vi "Find All Referenced Structures.vi"(8 "error in":errorcluster, 11 "ParseGDSII in":refnum<class "ParseGDSII.lvclass">) -> (0 "error out":errorcluster, 3 "ParseGDSII out":refnum<class "ParseGDSII.lvclass">)   [LabVIEW 2019, in "ParseGDSII.lvclass"]
uses:
  ParseGDSII.lvclass
  ParseGDSII.lvclass/ParseGDSII.ctl
  5fa63a74-4f9b-4856-8811-7cd17062abc4.vi
  DataTypes/Base/GDSII.DataType.lvclass
  Tree/Tree.lvclass
  Fast Tree/Fast Tree.lvclass
  920f742c-f628-416c-89cb-44049b089101.vi
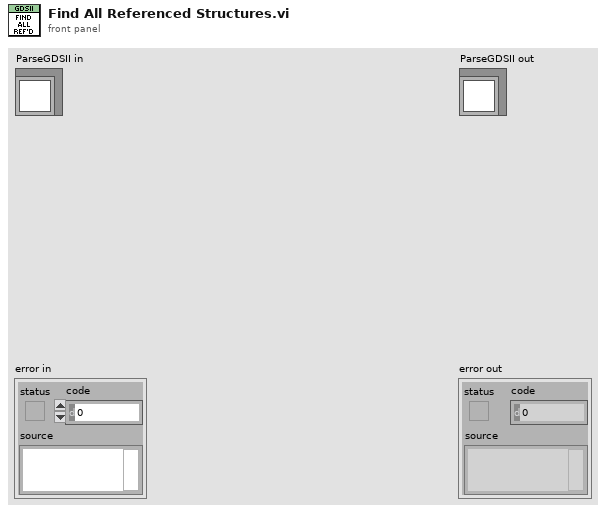
[diagram p1: front panel]
types:
  T1 = cluster{"Record Type":string, "Payload":string, "Parent Index":i32, "First Child Index":i32, "Next Sibling Index":i32}[]
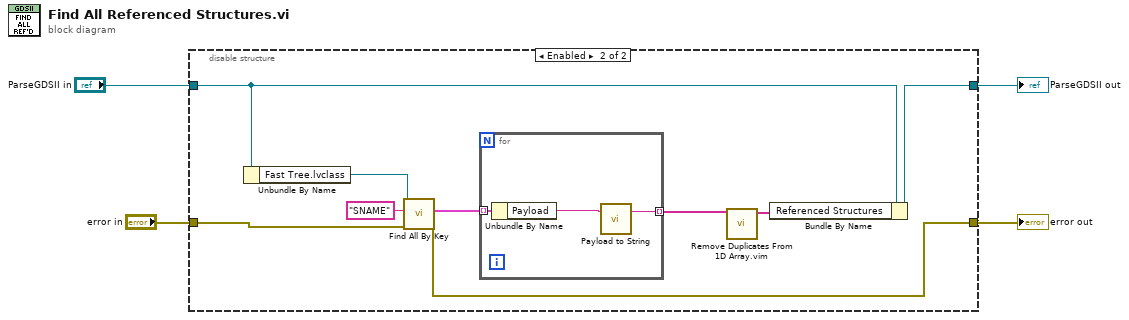
[diagram p0: block diagram]
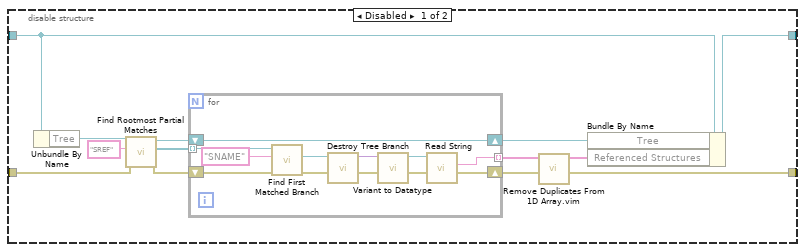
[diagram p2: hidden frame]
diagram:
  n1 = disable-structure shown="Enabled" {
    disable-tunnel: "error in" -> [w9 w28]
    disable-tunnel: [w8 w32] -> w3
    disable-tunnel: [w6 w30] -> w2
    disable-tunnel: "ParseGDSII in" -> [w5 w31]
    frame Disabled {
      n2 = Unbundle By Name(w5) -> ("Tree"=w12:refnum<class "Tree.lvclass">)
      n3 = call "Find Rootmost Partial Matches.vi"("error in"=w9, "Branch Name Pattern"="SREF", "Tree in"=w12) -> ("error out"=w10:errorcluster, "Root Most Partial Matches"=w14:refnum<class "Tree.lvclass">[], "Tree out"=w15:refnum<class "Tree.lvclass">)  [unwired: 5 in, 1 out]
      n4 = for {
        tunnel: w14 -> [w27] mode=indexing
        shift-right: [w22] -> w11
        shift-left: w15 -> [w22]
        tunnel: [w21] -> w13 mode=indexing
        shift-right: [w17] -> w8
        shift-left: w10 -> [w20]
        n5 = call "Find First Matched Branch.vi"("error in"=w20, "Branch Name Exact"="SNAME", "Tree in"=w27) -> ("error out"=w19:errorcluster, "Matched Branch"=w25:refnum<class "Tree.lvclass">)  [unwired: 5 in, 2 out]
        n6 = call "Destroy Tree Branch.vi"("error in"=w19, "Tree in"=w25) -> ("error out"=w18:errorcluster, "Root"=w24:variant)  [unwired: 8 in]
        n7 = call "Variant to Datatype.vi"("error in"=w18, "Variant"=w24) -> ("error out"=w17:errorcluster, "DataType"=w23:refnum<class "GDSII.DataType.lvclass">)  [unwired: 8 in]
        n8 = call-dynamic "Read String.vi"("GDSII.DataType in"=w23) -> ("String"=w21:string)  [unwired: 9 in, 1 out]
      }
      n9 = call "Remove Duplicates From 1D Array.vim"("array"=w13) -> ("array with duplicates removed"=w7:string[])  [unwired: 10 in]
      n10 = Bundle By Name(cluster=w5, "Tree"=w11, "Referenced Structures"=w7) -> (w6:refnum<class "ParseGDSII.lvclass">)
    }
    frame Enabled {
      n11 = Unbundle By Name(w31) -> ("Fast Tree.lvclass"=w35:refnum<class "Fast Tree.lvclass">)
      n12 = call "Find All By Key.vi"("error in"=w28, "Key"="SNAME", "Fast Tree in"=w35) -> ("error out"=w32:errorcluster, "Found Items"=w34:T1)  [unwired: 6 in, 1 out]
      n13 = for {
        tunnel: w34 -> [w39] mode=indexing
        tunnel: [w37] -> w33 mode=indexing
        n14 = Unbundle By Name(w39) -> ("Payload"=w38:string)
        n15 = call "Payload to String.vi"("Payload"=w38) -> ("String"=w37:string)  [unwired: 2 in]
      }
      n16 = call "Remove Duplicates From 1D Array.vim"("array"=w33) -> ("array with duplicates removed"=w29:string[])  [unwired: 10 in]
      n17 = Bundle By Name(cluster=w31, "Referenced Structures"=w29) -> (w30:refnum<class "ParseGDSII.lvclass">)
    }
  }
  "error out" <- w3
  "ParseGDSII out" <- w2
